vi "Neg Binomial CDF.vi"(9 "p":dbl=0.5, 10 "x":dbl=5.0, 11 "y":dbl) -> (0 "error":i32, 3 "cdf(y)":dbl=0.03125)   [LabVIEW 2018, in "NI_Gmath.lvlib"]
doc: "Computes the discrete cumulative distribution function (CDF), or the probability that the random variate X, where X describes the selected distribution type, takes on a value less than or equal to <B>x</B>. You must manually select the polymorphic instance to use."
uses:
  NI_Gmath.lvlib
  st_error_code.ctl
  Incomplete Beta Function.vi
panel:
  # "Negative Binomial CDF"
  # "failures"
  # "successes"
  # "probability"
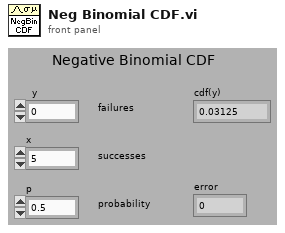
[diagram p1: front panel]
types:
  T1 = typedef "NI_Gmath.lvlib/st_error_code.ctl" = i32
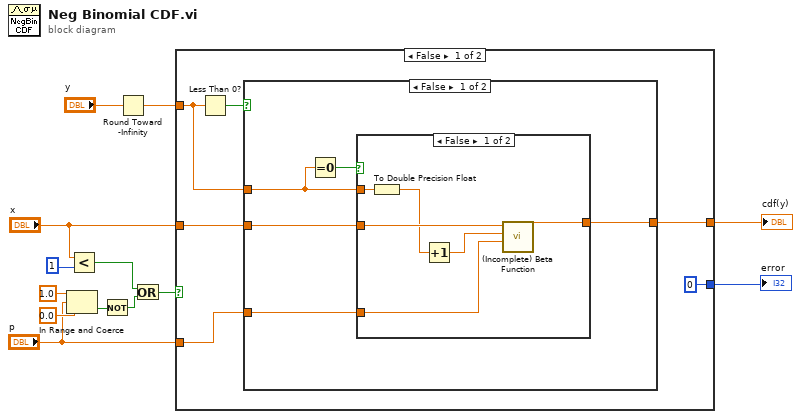
[diagram p0: block diagram]
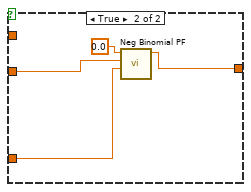
[diagram p2: hidden frame]
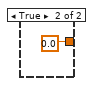
[diagram p3: hidden frame]
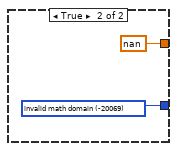
[diagram p4: hidden frame]
diagram:
  n1 = In Range and Coerce(upper limit=1.0, x="p", lower limit=0.0) -> (In Range?=w5:bool)  [unwired: 1 out]
  n2 = Less?(x="x", y=1) -> (x < y?=w3:bool)
  n3 = Not(x=w5) -> (.not. x?=w4:bool)
  n4 = Round Toward -Infinity(1:"y") -> (0:w1:dbl)
  n5 = Or(x=w3, y=w4) -> (x .or. y?=w8:bool)
  n6 = case shown="False" w8 {
    tunnel: [0 ("invalid math domain") w36] -> w13
    tunnel: [w18 nan] -> w12
    tunnel: w1 -> [w14 _]
    tunnel: "x" -> [w17 _]
    tunnel: "p" -> [w16 _]
    frame False {
      n7 = Less Than 0?(x=w14) -> (x < 0?=w15:bool)
      n8 = case shown="False" w15 {
        tunnel: [w24 0.0] -> w18
        tunnel: w14 -> [w23 _]
        tunnel: w17 -> [w22 _]
        tunnel: w16 -> [w21 _]
        frame False {
          n9 = Equal To 0?(x=w23) -> (x = 0?=w20:bool)
          n10 = case shown="False" w20 {
            tunnel: w22 -> [w28 w32]
            tunnel: w21 -> [w25 w33]
            tunnel: [w27 w31] -> w24
            tunnel: w23 -> [w30 _]
            frame False {
              n11 = To Double Precision Float(number=w30) -> (double precision float=w26:dbl)
              n12 = Increment(x=w26) -> (x+1=w29:dbl)
              n13 = call-poly "(Incomplete) Beta Function.vi"("a"=w25, "y"=w29, "x"=w28) -> ("b(x, y, a)"=w27:dbl)  [unwired: 8 in]
            }
            frame True {
              n14 = call "Neg Binomial PF.vi"("p"=w33, "x"=w32, "y"=0.0 ("a")) -> ("prob(y)"=w31:dbl)  [unwired: 7 in, 1 out]
            }
          }
        }
        frame True {
        }
      }
    }
    frame True {
      w36 = T1 -20069 items=["invalid math domain"=-20069, "Fourier interpolation size m >= n"=-20070, "empty array"=-20003] ("stat interp error code")
    }
  }
  "cdf(y)" <- w12
  "error" <- w13
